vi "GetOutputCount.vi"(7 "DLL path":path, 8 "error in (no error)":errorcluster, 11 "session id in":i32) -> (0 "error out":errorcluster, 2 "OutputCount":i32, 3 "session id out":i32)   [LabVIEW 2017, in "ONNX Class Library.lvlib"]
doc: "/**\n * @brief Получить количество выходов модели\n * \n * Возвращает число выходных тензоров, которые производит модель.\n * Модели классификации обычно имеют 1 выход, детекции объектов — несколько.\n * \n * @param sessionId [IN] ID сессии\n * \n * @return int32: Количество выходов (0 или больше)\n * @return int32: 0 если сессия не найдена или не загружена\n */\nint GetOutputCount(int sessionId);"
uses:
  ONNX Class Library.lvlib
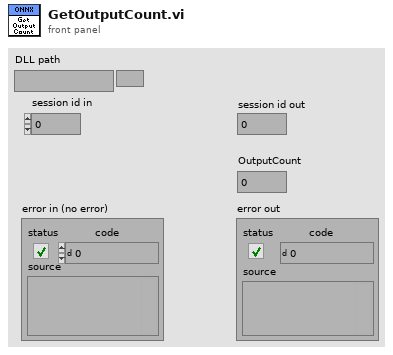
[diagram p1: front panel]
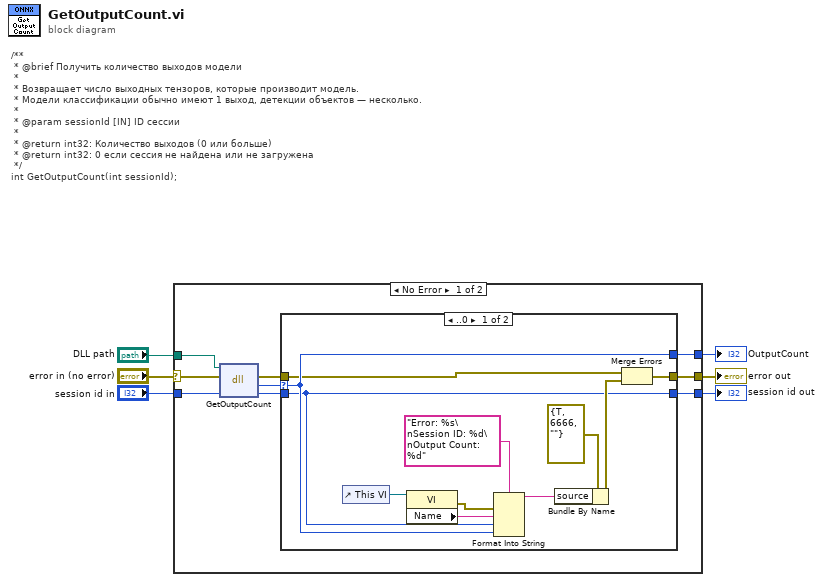
[diagram p0: block diagram]
diagram:
  # "/**\n * @brief Получить количество выходов модели\n * \n * Возвращает число выходных тензоров, которые производит модель.\n * Модели классификации обычно имеют 1 выход, детекции объектов — несколько.\n * \n * @param sessionId [IN] ID сессии\n * \n * @return int32: Количество выходов (0 или больше)\n * @return int32: 0 если сессия не найдена или не загружена\n */\nint GetOutputCount(int sessionId);"
  n1 = case shown="No Error" "error in (no error)" {
    selector: "error in (no error)" -> [w7 w31]
    tunnel: "session id in" -> [w15 w30]
    tunnel: [w11 _] -> w5
    tunnel: [w10 w31] -> w4
    tunnel: [w9 w30] -> w3
    tunnel: "DLL path" -> [w8 _]
    frame No Error {
      n2 = dll-call lib="home/ivan/LabVIEWData/ONNX/Test/libonnx_wrapper/unix64/libonnx_wrapper.so" fn="GetOutputCount"(path in=w8, error in=w7, "sessionId"=w15) -> (error out=w14:errorcluster, "return"=w13:i32, "sessionId"=w12:i32)  [unwired: 1 in, 1 out]
      n3 = case shown="..0" w13 {
        selector: w13 -> [w20 w27]
        tunnel: w14 -> [w16 w29]
        tunnel: [w17 w29] -> w10
        tunnel: w12 -> [w18 w28]
        tunnel: [w18 w28] -> w9
        tunnel: [w20 w27] -> w11
        frame ..0 {
          n4 = control-ref of="This VI"() -> (w23:refnum<vi>)
          n5 = property class="VI"(reference=w23) -> (error out=w19:errorcluster, "Name"=w22:string)  [unwired: 1 in, 1 out]
          n6 = Format Into String(format string="Error: %s\nSession ID: %d\nOutput Count: %d", error in=w19, w22, w18, w20) -> (resulting string=w24:string)  [unwired: 1 in, 1 out]
          n7 = Bundle By Name(cluster=errorcluster {"status"=TRUE, "code"=6666, "source"=""} ("error out"), "source"=w24) -> (w25:errorcluster)
          n8 = Merge Errors(w16, w25) -> (w17:errorcluster)
        }
        frame 1.. {
        }
      }
    }
    frame Error {
    }
  }
  "error out" <- w4
  "session id out" <- w3
  "OutputCount" <- w5
